vi "Write Registred Broadcast.vi"(8 "error in (no error)":errorcluster, 10 "Registred Broadcast":T1[](array[typedef]), 11 "Dqmh Module in":refnum<class "Dqmh Module.lvclass">) -> (0 "error out":errorcluster, 3 "Dqmh Module out":refnum<class "Dqmh Module.lvclass">)   [LabVIEW 2021, in "TAF Proj Document Type.lvlib" / "Dqmh Module.lvclass"]
uses:
  <vilib>/Wovalab/AntiDoc/Document Type/Add-ons/LabVIEW TAF Project/Dqmh Module/Dqmh Module.lvclass
  <vilib>/Wovalab/AntiDoc/Document Type/Add-ons/LabVIEW TAF Project/Dqmh Module/Module Broadcast Registred--cluster.ctl
  <vilib>/Wovalab/AntiDoc/Document Type/Add-ons/LabVIEW TAF Project/Dqmh Module/Dqmh Module.lvclass/Dqmh Module.ctl
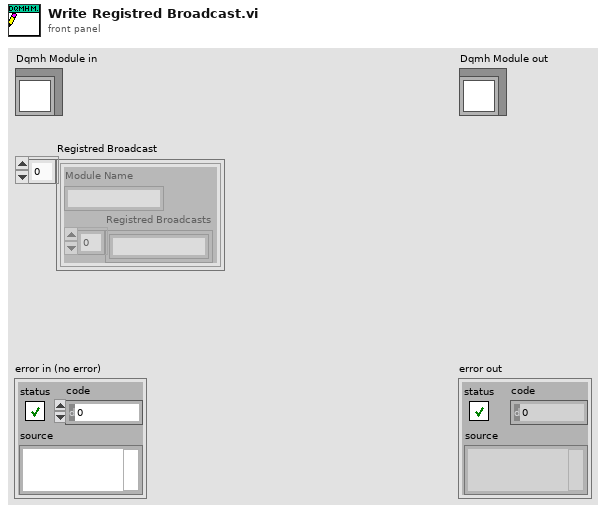
[diagram p1: front panel]
types:
  T1 = typedef "TAF Proj Document Type.lvlib/Dqmh Module.lvclass/Module Broadcast Registred--cluster.ctl" = cluster{"Module Name":string, "Registred Broadcasts":string[]}
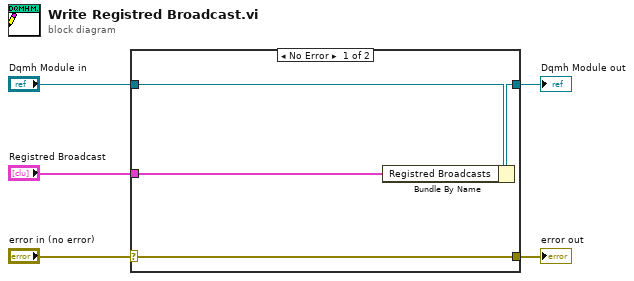
[diagram p0: block diagram]
diagram:
  n1 = case shown="No Error" "error in (no error)" {
    selector: "error in (no error)" -> [w9 w10]
    tunnel: [w9 w10] -> w4
    tunnel: [w7 w11] -> w2
    tunnel: "Dqmh Module in" -> [w8 w11]
    tunnel: "Registred Broadcast" -> [w6 _]
    frame No Error {
      n2 = Bundle By Name(cluster=w8, "Registred Broadcasts"=w6) -> (w7:refnum<class "Dqmh Module.lvclass">)
    }
    frame Error {
    }
  }
  "error out" <- w4
  "Dqmh Module out" <- w2
